vi "Pulse Train.vi"(6 "prototype spec":T1={"Prototype Pulse"=[], "delta t of Prototype Pulse (s) "=0.1}, 7 "interpolation method":i32(ring)=1 items=["Nearest", "Linear", "Spline", "Cubic Hermite"], 8 "Delay (s)":dbl[](array[numeric]), 9 "Amplitude":dbl[](array[numeric]), 10 "delta t of pulse train (s)":dbl=0.1, 11 "samples":i32=128) -> (0 "error":i32, 3 "Pulse Train":dbl[](array[numeric]))   [LabVIEW 2014, in "NI_AALBase.lvlib"]
doc: "Generates an array that concatenates a series of pulses according to the<B> Prototype Pulse</B>. This VI constructs the <B>Pulse Train</B> output by the specified <B>interpolation method</B>."
uses:
  NI_AALBase.lvlib
  Ramp Pattern by Samples.vi
panel:
  # "Pulse Train"
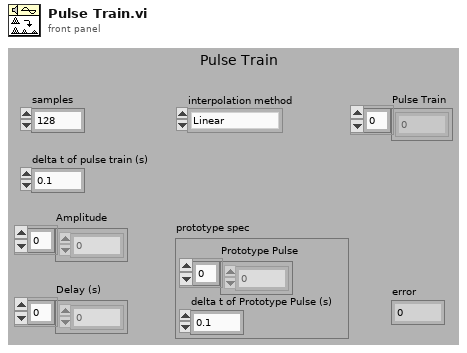
[diagram p1: front panel]
types:
  T1 = cluster{"Prototype Pulse":dbl[], "delta t of Prototype Pulse (s) ":dbl}
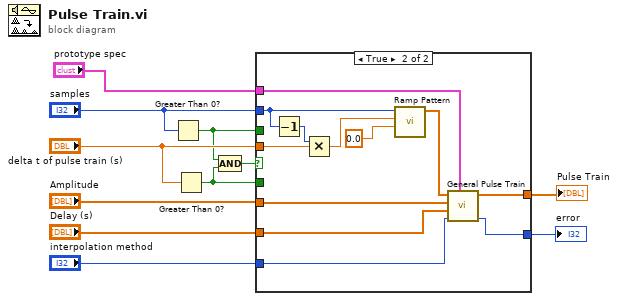
[diagram p0: block diagram]
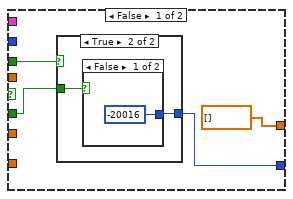
[diagram p2: hidden frame]
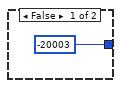
[diagram p3: hidden frame]
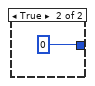
[diagram p4: hidden frame]
diagram:
  n1 = Greater Than 0?(x="samples") -> (x > 0?=w3:bool)
  n2 = Greater Than 0?(x="delta t of pulse train (s)") -> (x > 0?=w9:bool)
  n3 = Compound Arithmetic op=AND(w3, w9) -> (w10:bool)
  n4 = case shown="True" w10 {
    tunnel: "samples" -> [_ w29]
    tunnel: "delta t of pulse train (s)" -> [_ w28]
    tunnel: w9 -> [w12 _]
    tunnel: "prototype spec" -> [_ w24]
    tunnel: "interpolation method" -> [_ w23]
    tunnel: [dbl[] [] w27] -> w5
    tunnel: [w14 w26] -> w6
    tunnel: w3 -> [w13 _]
    tunnel: "Amplitude" -> [_ w22]
    tunnel: "Delay (s)" -> [_ w21]
    frame False {
      n5 = case shown="True" w13 {
        tunnel: [-20003 w18] -> w14
        tunnel: w12 -> [_ w17]
        frame False {
        }
        frame True {
          n6 = case shown="False" w17 {
            tunnel: [-20016 0] -> w18
            frame False {
            }
            frame True {
            }
          }
        }
      }
    }
    frame True {
      n7 = Decrement(x=w29) -> (x-1=w31:i32)
      n8 = Multiply(x=w31, y=w28) -> (x*y=w30:dbl)
      n9 = call-poly "Ramp Pattern.vi"("start"=0.0, "end"=w30, "samples"=w29) -> ("Ramp Pattern"=w25:dbl[])  [unwired: 7 in, 1 out]
      n10 = call "General Pulse Train.vi"("prototype spec"=w24, "method"=w23, "Delay"=w21, "Amplitude"=w22, "X"=w25) -> ("error"=w26:i32, "Pulse Train"=w27:dbl[])  [unwired: 5 in]
    }
  }
  "error" <- w6
  "Pulse Train" <- w5
